vi "MAIN_STANDALONE.vi"() -> ()   [LabVIEW 2019]
uses:
  LVPROJ_CONFIG_ESTACION/Type_defs/Coordenadas_estacion.ctl
  LVPROJ_CREAR BANDEJAS/Type_defs/Data_Bandeja.ctl
  TYPE'S DEF/OUTPUTS_TRASPASO_ASICS.ctl
  TYPE'S DEF/INPUT_TRASPASO_ASICS.ctl
  TYPE'S DEF/Estados_TRASPASO.ctl
  LVPROJ_MOVIMIENTO_CABEZAL/LABVIEW_MOVIMIENTO/MOVIMIENTO CABEZAL/Typedefs/Comandos.ctl
  LVPROJ_MOVIMIENTO_CABEZAL/LABVIEW_MOVIMIENTO/MOVIMIENTO CABEZAL/Typedefs/Estados_arduino.ctl
  LVPROJ_LEER_QR/LABVIEW/TYPE'S DEF/State_QR.ctl
  <vilib>/Instr/_visa.llb/VISA Configure Serial Port (Instr).vi
  SHARED VI'S/SHARED VI'S.lvlib
panel:
  out "trama datos devuelta":string
  out "trama datos enviada":string
  out "Asics pendientes":u32
  out "FINAL ASICS??":bool
  in  "Tab Control":T1(tab)
  in  "ENVIAR INPUTS TRASPASO":bool
  in  "EXIT":bool
  in  "COMENZAR TRASPASO":bool
  out "?":T2
  in  "DETENER TEST":bool
  out "PING OK":bool
  in  "TRASPASO ASICS INPUT":T3
  out "Configuracion Estación":T4={"Coordenadas_estacion"={"Coord.Bandeja entrada"={"Coord. X0 entrada"=0, "Coord. Y0 entrada "=0, "Altura Z entrada"=0}, "Coord.Bandeja OK"={"Coord. X0 OK"=0, "Coord. Y0 OK"=0, "Altura Z OK"=0}, "Coord.Bandeja entrada FAIL"={"Coord. X0 FAIL"=0, "Coord. Y0 FAIL"=0, "Altura Z FAIL"=0}, "Coord. Socket"={"Coord. X socket"=0, "Coord. Y socket"=0, "Altura Z socket"=0}}, "Nombre Bandeja"="", "Datos bandeja"={"Nº de columnas "=0, "Nº de filas "=0, "largo"=0, "ancho"=0, "nombre"="nombre", "Paso X (en mm)"=0.0, "Paso Y (en mm)"=0.0, "DISTANCIA SUELO A CHIP  "=0.0, "Nº de celdas totales"=0, "Distancia chips bandejas contiguas"=0.0}}
  out "Error Out":errorcluster
  in  "Error In":errorcluster
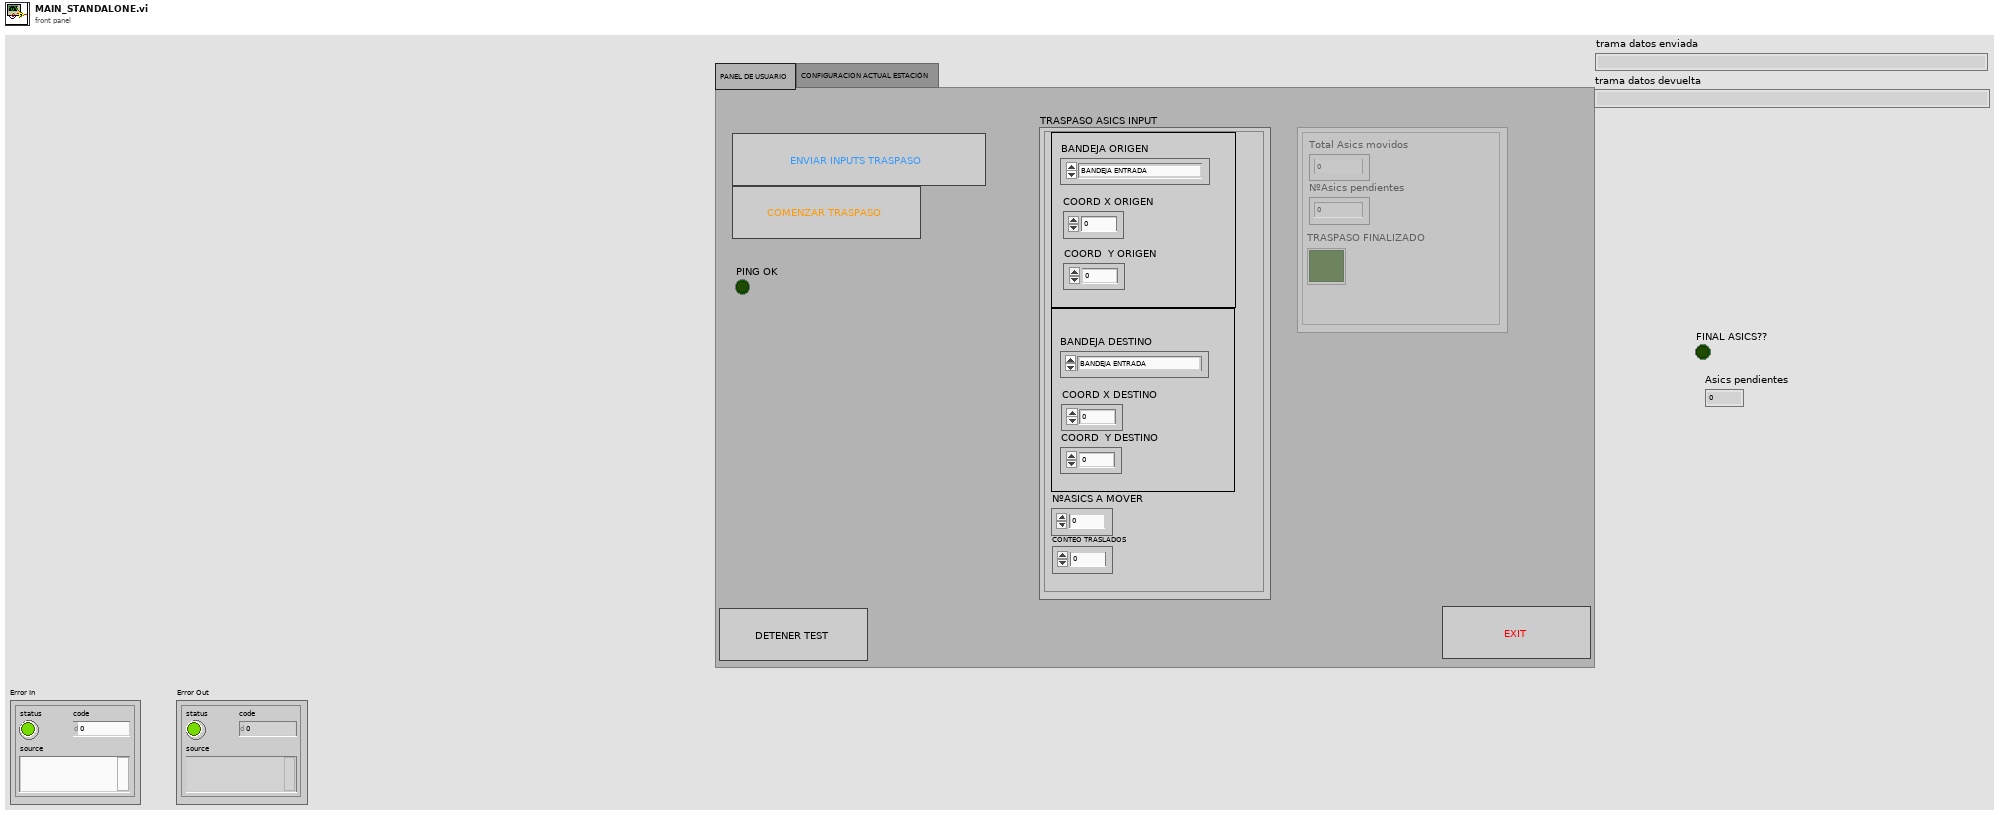
[diagram p1: front panel]
types:
  T1 = enum32{"PANEL DE USUARIO", "CONFIGURACION ACTUAL ESTACIÓN"}
  T2 = typedef "OUTPUTS_TRASPASO_ASICS.ctl" = cluster{"TRASPASO FINALIZADO":bool, "Total Asics movidos":u32, "NºAsics pendientes":u32}
  T3 = typedef "INPUT_TRASPASO_ASICS.ctl" = cluster{"COORD X ORIGEN":u32, "COORD  Y ORIGEN":u32, "NºASICS A MOVER":u32, "BANDEJA ORIGEN":enum16{"BANDEJA ENTRADA", "BANDEJA OK", "BANDEJA NOK"}, "BANDEJA DESTINO":enum16{"BANDEJA ENTRADA", "BANDEJA OK", "BANDEJA NOK"}, "COORD X DESTINO ":u32, "COORD  Y DESTINO ":u32, "CONTEO TRASLADOS":u32}
  T4 = typedef "Configuracion_estación.ctl" = cluster{"Coordenadas_estacion":T5, "Nombre Bandeja":string, "Datos bandeja":T6}
  T5 = typedef "Coordenadas_estacion.ctl" = cluster{"Coord.Bandeja entrada":cluster{"Coord. X0 entrada":u32, "Coord. Y0 entrada ":u32, "Altura Z entrada":u32}, "Coord.Bandeja OK":cluster{"Coord. X0 OK":u32, "Coord. Y0 OK":u32, "Altura Z OK":u32}, "Coord.Bandeja entrada FAIL":cluster{"Coord. X0 FAIL":u32, "Coord. Y0 FAIL":u32, "Altura Z FAIL":u32}, "Coord. Socket":cluster{"Coord. X socket":u32, "Coord. Y socket":u32, "Altura Z socket":u32}}
  T6 = typedef "Data_Bandeja.ctl" = cluster{"Nº de columnas ":u32, "Nº de filas ":u32, "largo":u32, "ancho":u32, "nombre":string, "Paso X (en mm)":dbl, "Paso Y (en mm)":dbl, "DISTANCIA SUELO A CHIP  ":dbl, "Nº de celdas totales":u16, "Distancia chips bandejas contiguas":dbl}
  T7 = typedef "Estados_TRASPASO.ctl" = enum16{"Init", "Wait for Event", "Init refs", "Init com", "Config estacion", "Introducir valores traspaso", "Home", "Ping_Arduino", "Esperar fin movimiento", "Enviar_config_test", "Actualizar valores", "Final traspaso?", "Terminar", "Exit", "Error?"}
  T8 = enum8{"Enabled", "Disabled", "Disabled and Grayed Out"}
  T9 = typedef "Estados_arduino.ctl" = enum16{"2", "3", "4", "5", "6", "7", "9", "8"}
  T10 = typedef "Comandos.ctl" = enum16{"H", "FH", "FM", "FI", "FX", "FY", "FZ", "I", "OK"}
  T11 = enum16{"BANDEJA ENTRADA", "BANDEJA OK", "BANDEJA NOK"}
  T12 = typedef "State_QR.ctl" = enum16{"Init", "Wait for Event", "Init refs", "Init com", "Config estacion", "Home", "Ping_Arduino", "Coge Asic", "Enviar_config_test", "Dejar Asic", "Leer QR", "Actualizar valores", "Enviar OK Arduino", "Final de lecturas?", "Terminar", "Exit", "Error?"}
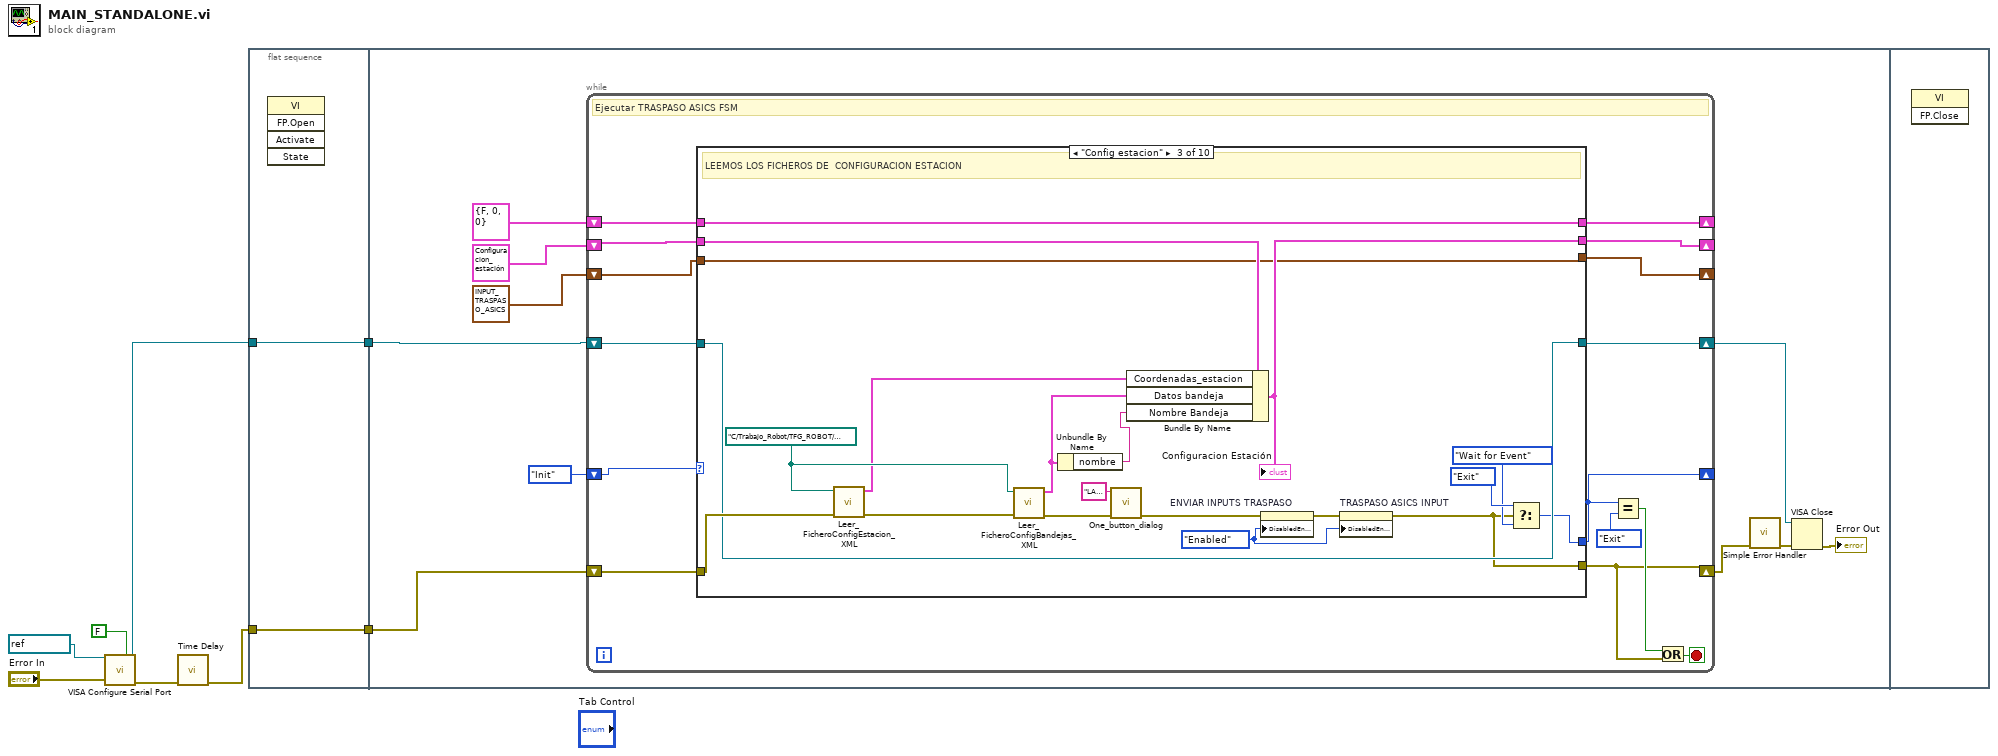
[diagram p0: block diagram]
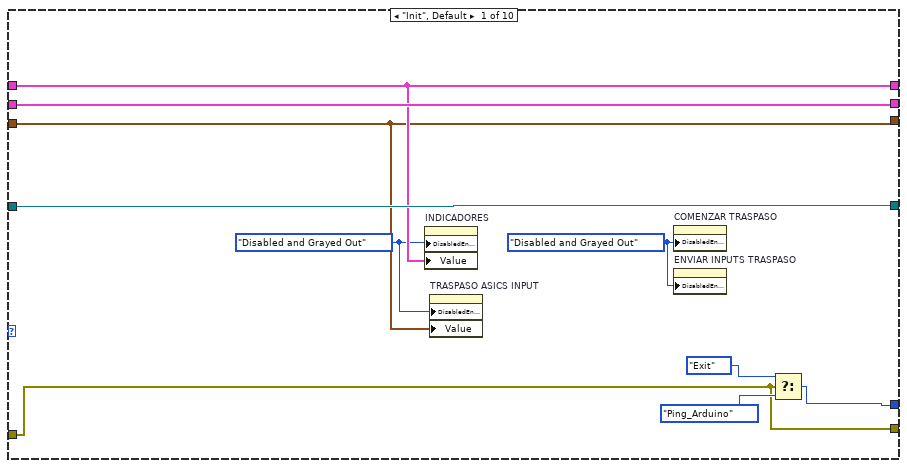
[diagram p2: hidden frame]
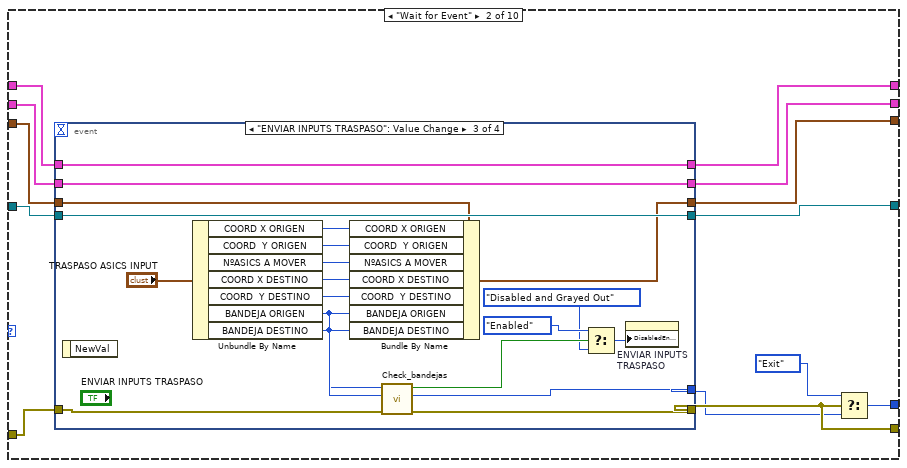
[diagram p3: hidden frame]
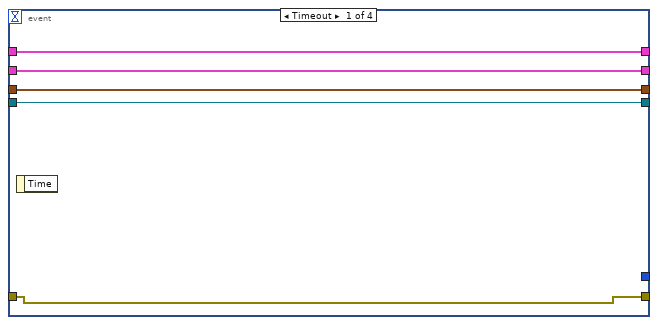
[diagram p4: hidden frame]
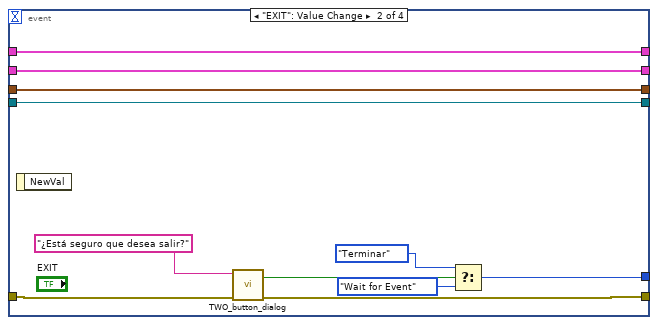
[diagram p5: hidden frame]
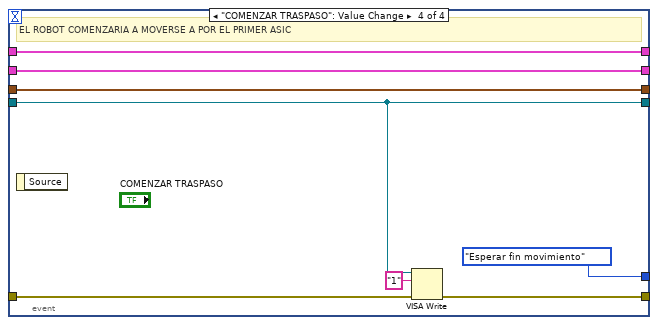
[diagram p6: hidden frame]
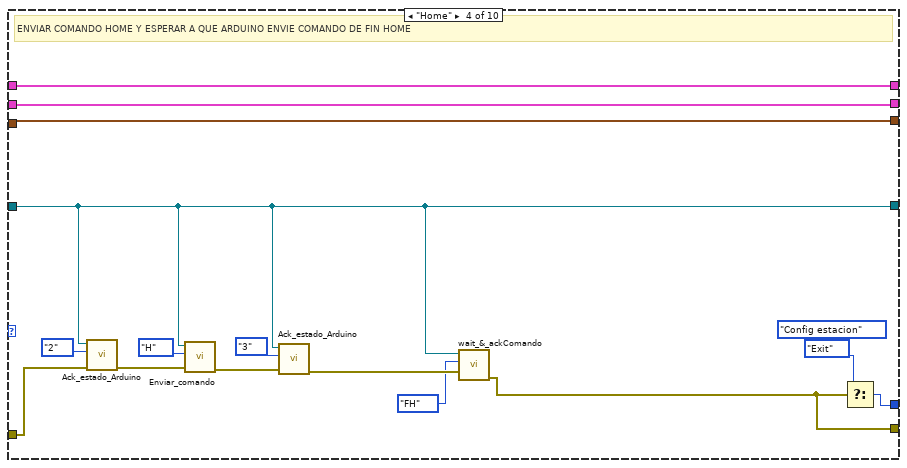
[diagram p7: hidden frame]
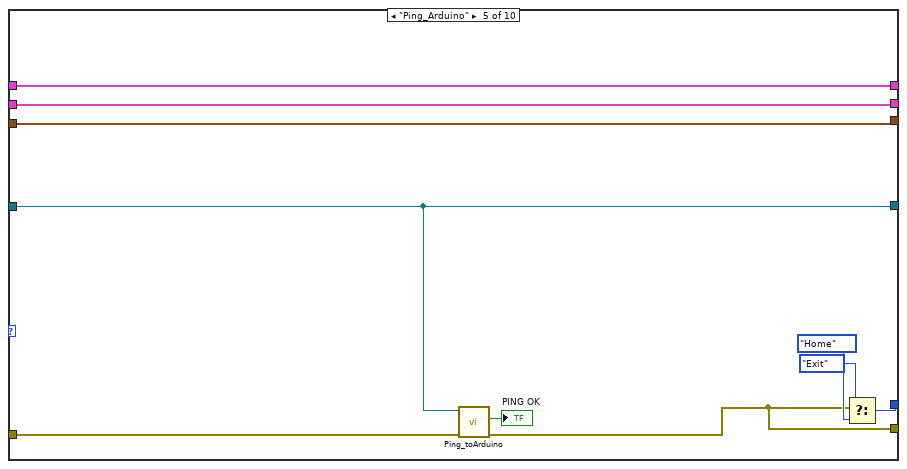
[diagram p8: hidden frame]
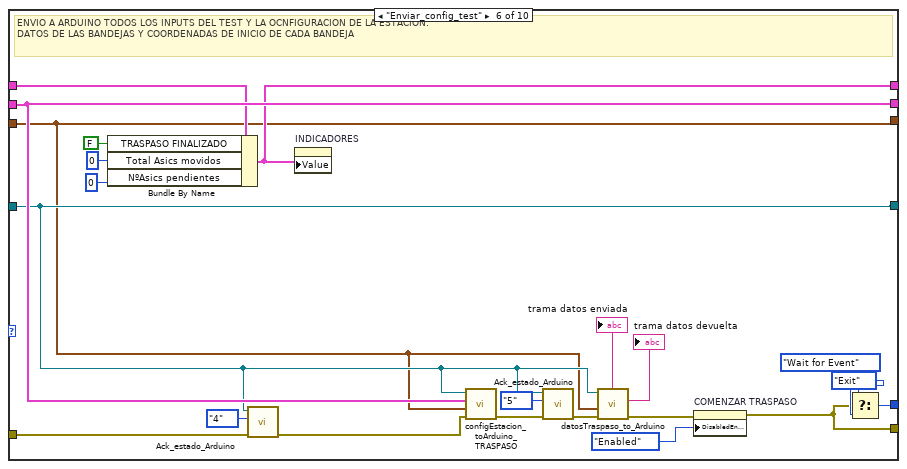
[diagram p9: hidden frame]
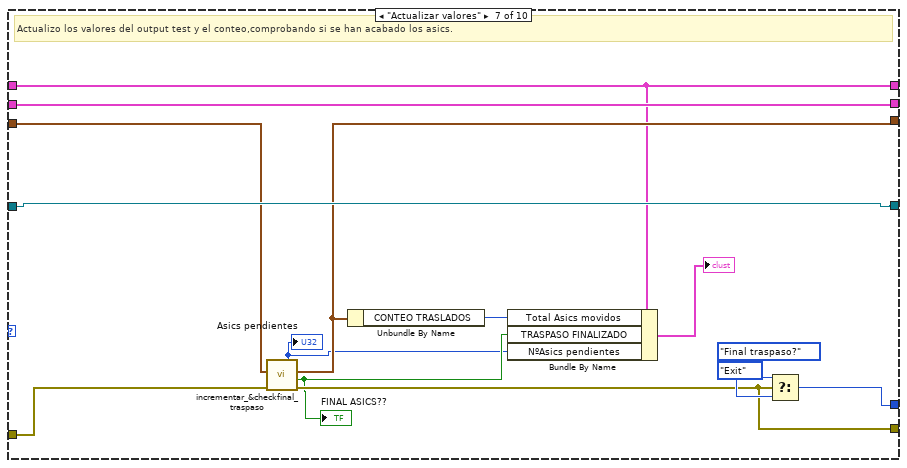
[diagram p10: hidden frame]
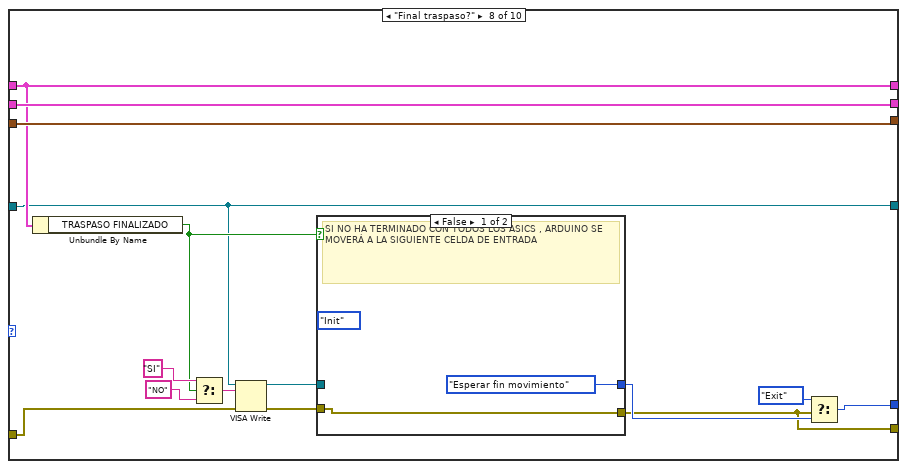
[diagram p11: hidden frame]
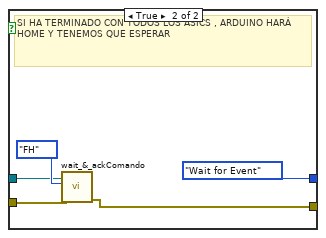
[diagram p12: hidden frame]
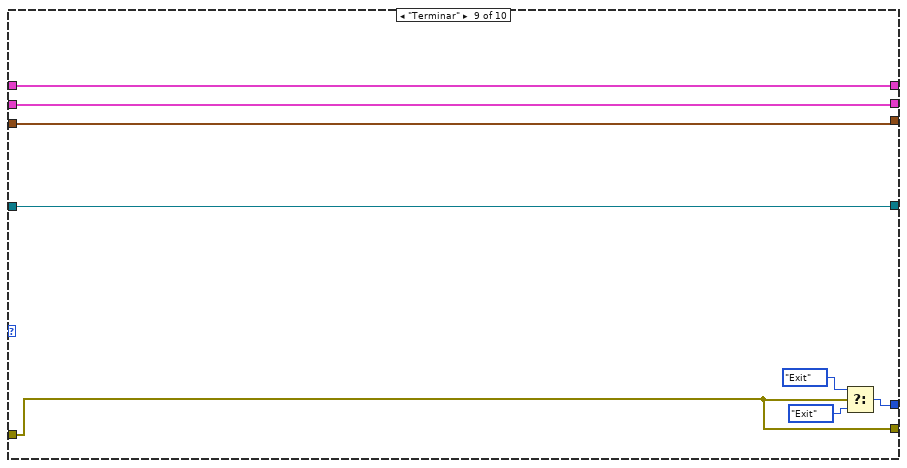
[diagram p13: hidden frame]
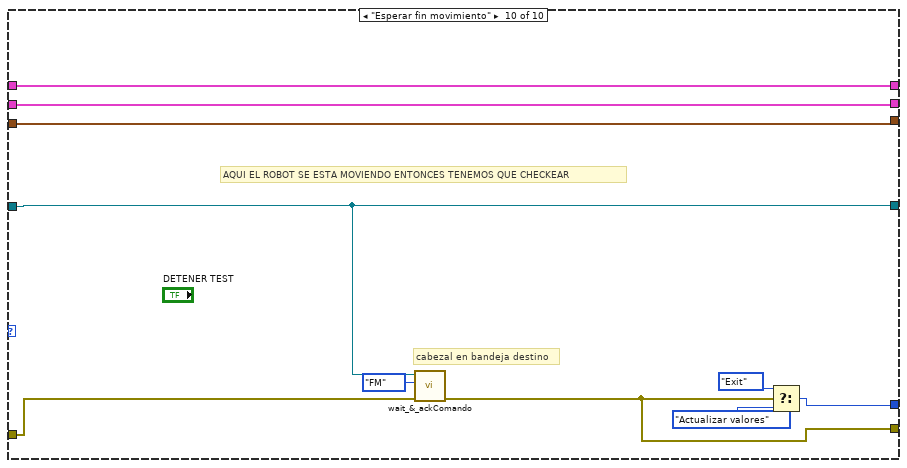
[diagram p14: hidden frame]
diagram:
  n1 = call-poly "VISA Configure Serial Port"("VISA resource name"=refnum<visa-resource-name> "COM4", "Enable Termination\nChar (T)"=FALSE ("Enable Termination\nChar (T)"), "error in (no error)"="Error In") -> ("VISA resource name out"=w1:refnum<visa-resource-name>, "error out"=w3:errorcluster)  [unwired: 11 in]
  n2 = call "Time Delay"("error in (no error)"=w3) -> ("error out"=w2:errorcluster)  [unwired: 10 in]
  n3 = flat-sequence {
    tunnel: w2 -> [w10]
    tunnel: [w10] -> w8
    tunnel: w1 -> [w9]
    tunnel: [w9] -> w7
    tunnel: w8 -> [w18]
    tunnel: w7 -> [w17]
    frame #0 {
      n4 = invoke class="VI" method="FP.Open"() -> ()  [unwired: 5 in, 5 out]
    }
    frame #1 {
      n5 = while {
        shift-right: [w30] -> w12
        shift-left: w18 -> [w34]
        shift-right: [w23] -> _
        shift-left: T3 {"COORD X ORIGEN"=0, "COORD  Y ORIGEN"=0, "NºASICS A MOVER"=1, "BANDEJA ORIGEN"=enum."BANDEJA ENTRADA", "BANDEJA DESTINO"=enum."BANDEJA OK", "COORD X DESTINO "=0, "COORD  Y DESTINO "=0, "CONTEO TRASLADOS"=0} ("TEST ASICS INPUT") -> [w33]
        shift-right: [w25] -> _
        shift-left: T4 {"Coordenadas_estacion"={"Coord.Bandeja entrada"={"Coord. X0 entrada"=0, "Coord. Y0 entrada "=0, "Altura Z entrada"=0}, "Coord.Bandeja OK"={"Coord. X0 OK"=0, "Coord. Y0 OK"=0, "Altura Z OK"=0}, "Coord.Bandeja entrada FAIL"={"Coord. X0 FAIL"=0, "Coord. Y0 FAIL"=0, "Altura Z FAIL"=0}, "Coord. Socket"={"Coord. X socket"=0, "Coord. Y socket"=0, "Altura Z socket"=0}}, "Nombre Bandeja"="", "Datos bandeja"={"Nº de columnas "=0, "Nº de filas "=0, "largo"=0, "ancho"=0, "nombre"="nombre", "Paso X (en mm)"=0.0, "Paso Y (en mm)"=0.0, "DISTANCIA SUELO A CHIP  "=0.0, "Nº de celdas totales"=0, "Distancia chips bandejas contiguas"=0.0}} ("Configuracion Estación") -> [w29]
        shift-right: [w27] -> w13
        shift-left: w17 -> [w28]
        shift-right: [w24] -> _
        shift-left: T2 {"TRASPASO FINALIZADO"=FALSE, "Total Asics movidos"=0, "NºAsics pendientes"=0} -> [w26]
        shift-right: [w21] -> _
        shift-left: Estados_TRASPASO."Init" ("States_main") -> [w22]
        stop <- w32 stop-if-true
        # "Ejecutar TRASPASO ASICS FSM"
        n6 = case shown="\"Config estacion\"" w22 {
          tunnel: w34 -> [w41 w52 w122 w129 w142 w168 w179 w190 w210 w221]
          tunnel: w33 -> [w36 w54 w111 w136 w146 w149 w177 w196 w212 w220]
          tunnel: [w41 w51 w104 w124 w141 w154 w178 w185 w210 w217] -> w30
          tunnel: w29 -> [w43 w56 w114 w137 w147 w167 w182 w197 w213 w219]
          tunnel: w28 -> [w42 w49 w115 w126 w140 w161 w181 w189 w211 w216]
          tunnel: [w42 w48 w115 w126 w140 w161 w181 w189 w211 w216] -> w27
          tunnel: w26 -> [w39 w58 w112 w138 w148 w159 w173 w195 w214 w218]
          tunnel: [w43 w55 w113 w137 w147 w167 w182 w197 w213 w219] -> w25
          tunnel: [w39 w57 w112 w138 w148 w150 w173 w195 w214 w218] -> w24
          tunnel: [w36 w53 w111 w136 w146 w149 w175 w196 w212 w220] -> w23
          tunnel: [w40 w46 w108 w123 w143 w165 w180 w198 w207 w222] -> w21
          frame "Init", Default {
            w38 = T8."Disabled and Grayed Out" ("Disabled")
            w37 = T8."Disabled and Grayed Out" ("Disabled")
            n7 = property on="INDICADORES" class="Clust (strict)"("DisabledEnum"=w37, "Value"=w39) -> ()  [unwired: 2 in, 2 out]
            n8 = property on="TRASPASO ASICS INPUT" class="Clust (strict)"("DisabledEnum"=w37, "Value"=w36) -> ()  [unwired: 2 in, 2 out]
            n9 = property on="COMENZAR TRASPASO" class="Bool"("DisabledEnum"=w38) -> ()  [unwired: 2 in, 2 out]
            n10 = property on="ENVIAR INPUTS TRASPASO" class="Bool"("DisabledEnum"=w38) -> ()  [unwired: 2 in, 2 out]
            n11 = Select(t=Estados_TRASPASO."Exit" ("States_main"), s=w41, f=Estados_TRASPASO."Ping_Arduino" ("States_main")) -> (s? t:f=w40:T7)
          }
          frame "Wait for Event" {
            n12 = event shown="[2] \"ENVIAR INPUTS TRASPASO\": Value Change" {
              selector: _ -> [_ _ _ _]
              dyn-events: _ -> [_ _ _ _]
              timeout: _ -> [_ _ _ _]
              tunnel: w58 -> [w63 w74 w94 w102]
              tunnel: [w63 w74 w94 w102] -> w57
              tunnel: w56 -> [w62 w73 w93 w101]
              tunnel: [w62 w73 w93 w101] -> w55
              tunnel: w54 -> [w61 w72 w85 w100]
              tunnel: [w61 w72 w84 w100] -> w53
              tunnel: w52 -> [w60 w71 w81 w98]
              tunnel: [w60 w69 w75 w97] -> w51
              tunnel: w49 -> [w59 w70 w92 w99]
              tunnel: [w59 w70 w92 w99] -> w48
              tunnel: [_ w64 w80 Estados_TRASPASO."Esperar fin movimiento" ("States_main")] -> w47
              event Timeout {
                n13 = event-data() -> ()  [unwired: 1 in, 1 out]
              }
              event "EXIT": Value Change {
                n14 = event-data() -> ()  [unwired: 1 in, 1 out]
                n15 = call "TWO_button_dialog.vi"("error in (no error)"=w71, "message"="¿Está seguro que desea salir?") -> ("error out"=w69:errorcluster, "si/no"=w67:bool)  [unwired: 8 in]
                n16 = Select(t=Estados_TRASPASO."Terminar" ("States_main"), s=w67, f=Estados_TRASPASO."Wait for Event") -> (s? t:f=w64:T7)
              }
              event "ENVIAR INPUTS TRASPASO": Value Change {
                n17 = event-data() -> ()  [unwired: 1 in, 1 out]
                n18 = Unbundle By Name("TRASPASO ASICS INPUT") -> ("COORD X ORIGEN"=w90:u32, "COORD  Y ORIGEN"=w89:u32, "NºASICS A MOVER"=w88:u32, "COORD X DESTINO"=w87:u32, "COORD  Y DESTINO"=w86:u32, "BANDEJA ORIGEN"=w83:T11, "BANDEJA DESTINO"=w82:T11)
                n19 = Bundle By Name(cluster=w85, "COORD X ORIGEN"=w90, "COORD  Y ORIGEN"=w89, "NºASICS A MOVER"=w88, "COORD X DESTINO"=w87, "COORD  Y DESTINO"=w86, "BANDEJA ORIGEN"=w83, "BANDEJA DESTINO"=w82) -> (w84:T3)
                n20 = call "Check_bandejas.vi"("error in (no error)"=w81, "BANDEJA ORIGEN"=w83, "BANDEJA DESTINO"=w82) -> ("error out"=w75:errorcluster, "States_main"=w80:T7, "Datos incorrectos"=w79:bool)  [unwired: 6 in]
                n21 = Select(t=T8."Enabled" ("Disabled"), s=w79, f=T8."Disabled and Grayed Out") -> (s? t:f=w76:T8)
                n22 = property on="ENVIAR INPUTS TRASPASO" class="Bool"("DisabledEnum"=w76) -> ()  [unwired: 2 in, 2 out]
              }
              event "COMENZAR TRASPASO": Value Change {
                # "EL ROBOT COMENZARIA A MOVERSE A POR EL PRIMER ASIC"
                n23 = event-data() -> ()  [unwired: 1 in, 1 out]
                n24 = VISA Write(VISA resource name=w99, write buffer="1", error in (no error)=w98) -> (error out=w97:errorcluster)  [unwired: 2 out]
              }
            }
            n25 = Select(t=Estados_TRASPASO."Exit" ("States_main"), s=w51, f=w47) -> (s? t:f=w46:T7)
          }
          frame "Config estacion" {
            w103 = T8."Enabled" ("Disabled")
            w120 = path "C:/Trabajo_Robot/TFG_ROBOT/CONTROL_ROBOT/LABVIEW_ROBOT_MASTER" ("XML File Path")
            # "LEEMOS LOS FICHEROS DE  CONFIGURACION ESTACION"
            n26 = call "Leer_FicheroConfigEstacion_XML.vi"("error in (no error)"=w122, "XML File Path"=w120) -> ("error out"=w121:errorcluster, "Coordenadas_estacion"=w119:T5)  [unwired: 8 in]
            n27 = call "Leer_FicheroConfigBandejas_XML.vi"("error in (no error)"=w121, "XML File Path"=w120) -> ("error out"=w116:errorcluster, "Datos bandeja"=w118:T6)  [unwired: 8 in]
            n28 = Unbundle By Name(w118) -> ("nombre"=w117:string)
            n29 = call "One_button_dialog.vi"("error in (no error)"=w116, "message"="LA CONFIGURACION DE LA ESTACIÓN SE HA LEÍDO CORRECTAMENTE") -> ("error out"=w106:errorcluster)  [unwired: 9 in]
            n30 = Bundle By Name(cluster=w114, "Coordenadas_estacion"=w119, "Datos bandeja"=w118, "Nombre Bandeja"=w117) -> (w113:T4)
            "Configuracion Estación" <- w113
            n31 = property on="ENVIAR INPUTS TRASPASO" class="Bool"(error in=w106, "DisabledEnum"=w103) -> (error out=w105:errorcluster)  [unwired: 1 in, 1 out]
            n32 = property on="TRASPASO ASICS INPUT" class="Clust (strict)"(error in=w105, "DisabledEnum"=w103) -> (error out=w104:errorcluster)  [unwired: 1 in, 1 out]
            n33 = Select(t=Estados_TRASPASO."Exit" ("States_main"), s=w104, f=Estados_TRASPASO."Wait for Event" ("States_main")) -> (s? t:f=w108:T7)
          }
          frame "Home" {
            # "ENVIAR COMANDO HOME Y ESPERAR A QUE ARDUINO ENVIE COMANDO DE FIN HOME"
            n34 = call "Ack_estado_Arduino.vi"("error in (no error)"=w129, "Enum"=Estados_arduino."2", "VISA resource name"=w126) -> ("error out"=w135:errorcluster)  [unwired: 6 in, 2 out]
            n35 = call "Enviar_comando.vi"("error in (no error)"=w135, "Enum"=Comandos."H", "VISA resource name"=w126) -> ("error out"=w130:errorcluster)  [unwired: 6 in, 2 out]
            n36 = call "Ack_estado_Arduino.vi"("error in (no error)"=w130, "Enum"=Estados_arduino."3", "VISA resource name"=w126) -> ("error out"=w131:errorcluster)  [unwired: 6 in, 2 out]
            n37 = call "wait_&_ackComando.vi"("error in (no error)"=w131, 10:Comandos."FH", "VISA Refnum in"=w126) -> ("error out"=w124:errorcluster)  [unwired: 7 in, 1 out]
            n38 = Select(t=Estados_TRASPASO."Exit" ("States_main"), s=w124, f=Estados_TRASPASO."Config estacion" ("States_main")) -> (s? t:f=w123:T7)
          }
          frame "Ping_Arduino" {
            n39 = call "Ping_toArduino.vi"("error in (no error)"=w142, "VISA Refnum in"=w140) -> ("error out"=w141:errorcluster, "PING OK"=→"PING OK":bool)  [unwired: 7 in, 1 out]
            n40 = Select(t=Estados_TRASPASO."Exit" ("States_main"), s=w141, f=Estados_TRASPASO."Home" ("States_main")) -> (s? t:f=w143:T7)
          }
          frame "Enviar_config_test" {
            # "ENVIO A ARDUINO TODOS LOS INPUTS DEL TEST Y LA OCNFIGURACION DE LA ESTACIÓN:\nDATOS DE LAS BANDEJAS Y COORDENADAS DE INICIO DE CADA BANDEJA"
            n41 = Bundle By Name(cluster=w159, "TRASPASO FINALIZADO"=FALSE, "Total Asics movidos"=u32 0, "NºAsics pendientes"=u32 0) -> (w150:T2)
            n42 = call "Ack_estado_Arduino.vi"("error in (no error)"=w168, "Enum"=Estados_arduino."4", "VISA resource name"=w161) -> ("error out"=w164:errorcluster)  [unwired: 6 in, 2 out]
            n43 = property on="INDICADORES" class="Clust (strict)"("Value"=w150) -> ()  [unwired: 2 in, 2 out]
            n44 = call "configEstacion_toArduino_TRASPASO.vi"("error in (no error)"=w164, "TRASPASO ASICS INPUT"=w149, "Configuracion Estación"=w167, "VISA resource name"=w161) -> ("error IO"=w166:errorcluster)  [unwired: 5 in, 2 out]
            n45 = call "Ack_estado_Arduino.vi"("error in (no error)"=w166, "Enum"=Estados_arduino."5", "VISA resource name"=w161) -> ("error out"=w163:errorcluster)  [unwired: 6 in, 2 out]
            n46 = call "datosTraspaso_to_Arduino.vi"("error in (no error)"=w163, "TRASPASO ASICS INPUT"=w149, "VISA resource name"=w161) -> ("error IO"=w155:errorcluster, "trama datos devuelta"=→"trama datos devuelta":string, "trama datos enviada"=→"trama datos enviada":string)  [unwired: 6 in]
            n47 = property on="COMENZAR TRASPASO" class="Bool"(error in=w155, "DisabledEnum"=T8."Enabled" ("Disabled")) -> (error out=w154:errorcluster)  [unwired: 1 in, 1 out]
            n48 = Select(t=Estados_TRASPASO."Exit" ("States_main"), s=w154, f=Estados_TRASPASO."Wait for Event" ("States_main")) -> (s? t:f=w165:T7)
          }
          frame "Actualizar valores" {
            # "Actualizo los valores del output test y el conteo,comprobando si se han acabado los asics."
            n49 = call "incrementar_&checkfinal_traspaso.vi"("error in (no error)"=w179, "TRASPASO ASICS INPUT"=w177) -> ("error out"=w178:errorcluster, "FINAL ASICS??"=w174:bool, "output cluster"=w175:T3, "Asics pendientes"=w171:u32)  [unwired: 6 in]
            "FINAL ASICS??" <- w174
            "Asics pendientes" <- w171
            n50 = Unbundle By Name(w175) -> ("CONTEO TRASLADOS"=w176:u32)
            n51 = Bundle By Name(cluster=w173, "Total Asics movidos"=w176, "TRASPASO FINALIZADO"=w174, "NºAsics pendientes"=w171) -> (→"?":T2)
            n52 = Select(t=Estados_TRASPASO."Exit" ("States_main"), s=w178, f=Estados_TRASPASO."Final traspaso?" ("States_main")) -> (s? t:f=w180:T7)
          }
          frame "Final traspaso?" {
            (unwired) State_QR."Init" ("States_main")
            n53 = Unbundle By Name(w195) -> ("TRASPASO FINALIZADO"=w191:bool)
            n54 = Select(t="SI", s=w191, f="NO") -> (s? t:f=w192:string)
            n55 = VISA Write(VISA resource name=w189, write buffer=w192, error in (no error)=w190) -> (VISA resource name out=w186:refnum<visa-resource-name>, error out=w188:errorcluster)  [unwired: 1 out]
            n56 = case shown="False" w191 {
              tunnel: w188 -> [w200 w205]
              tunnel: [Estados_TRASPASO."Esperar fin movimiento" ("States_main") Estados_TRASPASO."Wait for Event" ("States_main")] -> w187
              tunnel: [w200 w203] -> w185
              tunnel: w186 -> [_ w202]
              frame False {
                # "SI NO HA TERMINADO CON TODOS LOS ASICS , ARDUINO SE MOVERÁ A LA SIGUIENTE CELDA DE ENTRADA"
              }
              frame True {
                # "SI HA TERMINADO CON TODOS LOS ASICS , ARDUINO HARÁ HOME Y TENEMOS QUE ESPERAR"
                n57 = call "wait_&_ackComando.vi"("error in (no error)"=w205, 10:Comandos."FH", "VISA Refnum in"=w202) -> ("error out"=w203:errorcluster)  [unwired: 7 in, 1 out]
              }
            }
            n58 = Select(t=Estados_TRASPASO."Exit" ("States_main"), s=w185, f=w187) -> (s? t:f=w198:T7)
          }
          frame "Terminar" {
            n59 = Select(t=Estados_TRASPASO."Exit" ("y"), s=w210, f=Estados_TRASPASO."Exit" ("y")) -> (s? t:f=w207:T7)
          }
          frame "Esperar fin movimiento" {
            # "cabezal en bandeja destino"
            # "AQUI EL ROBOT SE ESTA MOVIENDO ENTONCES TENEMOS QUE CHECKEAR"
            n60 = call "wait_&_ackComando.vi"("error in (no error)"=w221, 10:Comandos."FM", "VISA Refnum in"=w216) -> ("error out"=w217:errorcluster)  [unwired: 7 in, 1 out]
            n61 = Select(t=Estados_TRASPASO."Exit" ("States_main"), s=w217, f=Estados_TRASPASO."Actualizar valores" ("States_main")) -> (s? t:f=w222:T7)
          }
        }
        n62 = Equal?(x=w21, y=Estados_TRASPASO."Exit") -> (x = y?=w35:bool)
        n63 = Or(x=w35, y=w30) -> (x .or. y?=w32:bool)
      }
      n64 = call <vilib>:"Simple Error Handler.vi"("error in (no error)"=w12) -> ("error out"=w11:errorcluster)  [unwired: 4 in, 4 out]
      n65 = VISA Close(VISA resource name=w13, error in (no error)=w11) -> (error out=→"Error Out":errorcluster)
    }
    frame #2 {
      n66 = invoke class="VI" method="FP.Close"() -> ()  [unwired: 3 in, 3 out]
    }
  }
